vi "Rysuj Wielościan.vi"(0 "tablica punktów":dbl[][](array[numeric]), 1 "Środek":dbl[](array[numeric]), 2 "przeskalowanie":i32, 3 "color":u32(colorbox), 4 "przed rysunkiem":picture) -> (5 "po rysunku":picture)   [LabVIEW 2016]
doc: "To vi rysuje wielokąt o wierzchołka z tablicy 2d (wektory względem przekazanego środka) i wypełnia zadanym kolorem"
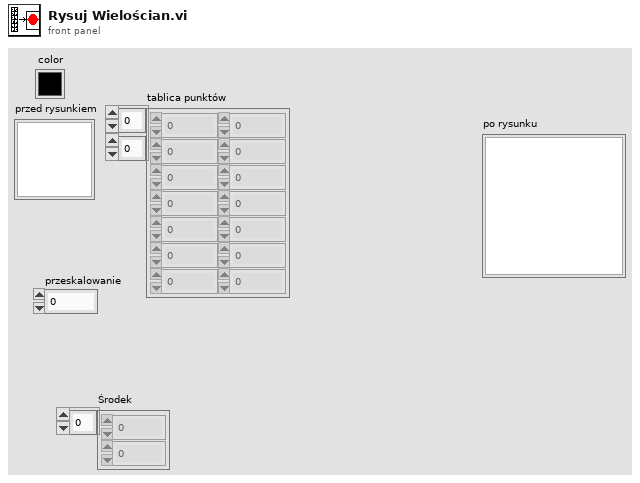
[diagram p1: front panel]
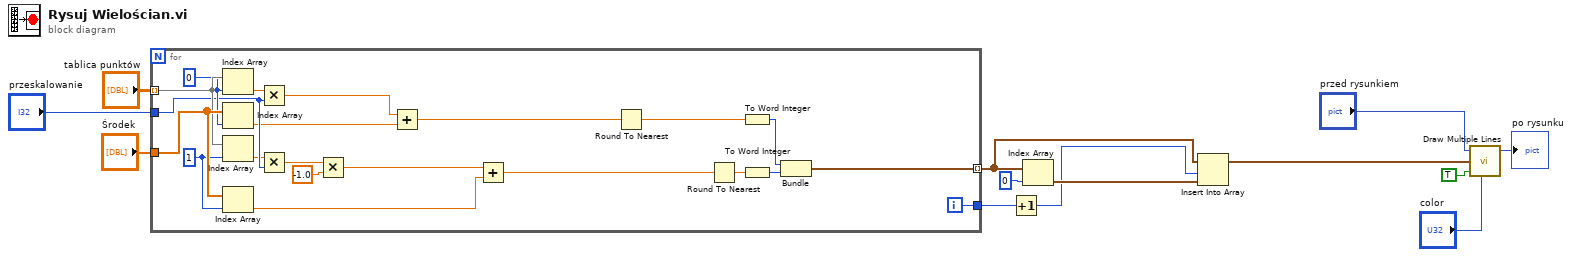
[diagram p0: block diagram]
diagram:
  n1 = for {
    tunnel: "tablica punktów" -> [w33] mode=indexing
    tunnel: "Środek" -> [w34]
    tunnel: "przeskalowanie" -> [w30]
    tunnel: [w24] -> w6 mode=indexing
    tunnel: [w17] -> w5
    i -> [w17]
    w31 = 1 ("index")
    w32 = 0 ("index")
    n2 = Index Array(array=w33, index=w32) -> (element=w29:dbl)
    n3 = Index Array(array=w34, index=w32) -> (element=w26:dbl)
    n4 = Index Array(array=w33, index=w31) -> (element=w28:dbl)
    n5 = Index Array(array=w34, index=w31) -> (element=w25:dbl)
    n6 = Multiply(x=w29, y=w30) -> (x*y=w27:dbl)
    n7 = Multiply(x=w28, y=w30) -> (x*y=w15:dbl)
    n8 = Multiply(x=w15, y=-1.0) -> (x*y=w14:dbl)
    n9 = Add(x=w27, y=w26) -> (x+y=w23:dbl)
    n10 = Add(x=w14, y=w25) -> (x+y=w21:dbl)
    n11 = Round To Nearest(number=w23) -> (nearest integer value=w22:dbl)
    n12 = Round To Nearest(number=w21) -> (nearest integer value=w20:dbl)
    n13 = To Word Integer(number=w22) -> (16bit integer=w19:i16)
    n14 = To Word Integer(number=w20) -> (16bit integer=w18:i16)
    n15 = Bundle(w19, w18) -> (w24:cluster{i16, i16})  [unwired: 1 in]
  }
  n16 = Increment(x=w5) -> (x+1=w4:i32)
  n17 = Index Array(array=w6, index=0) -> (element=w7:cluster{i16, i16})
  n18 = Insert Into Array(array=w6, index=w4, new element=w7) -> (w3:cluster{i16, i16}[])
  n19 = call <vilib>:"Draw Multiple Lines.vi"("picture"="przed rysunkiem", "line endpoints"=w3, "fill?(F)"=TRUE, "color(black)"="color") -> ("new picture"=→"po rysunku":picture)  [unwired: 5 in]
